vi "PSConverter.vi"(1 "Tbl Refnum":refnum<vi>, 2 "PROC":string[](array[string]), 3 "STATES":string[][](array[string]), 4 "Input claster":cluster{"TimeInState":u16, "cur_state":i8}[](array[cluster])) -> (0 "Current States":string[][](table))   [LabVIEW 2019]
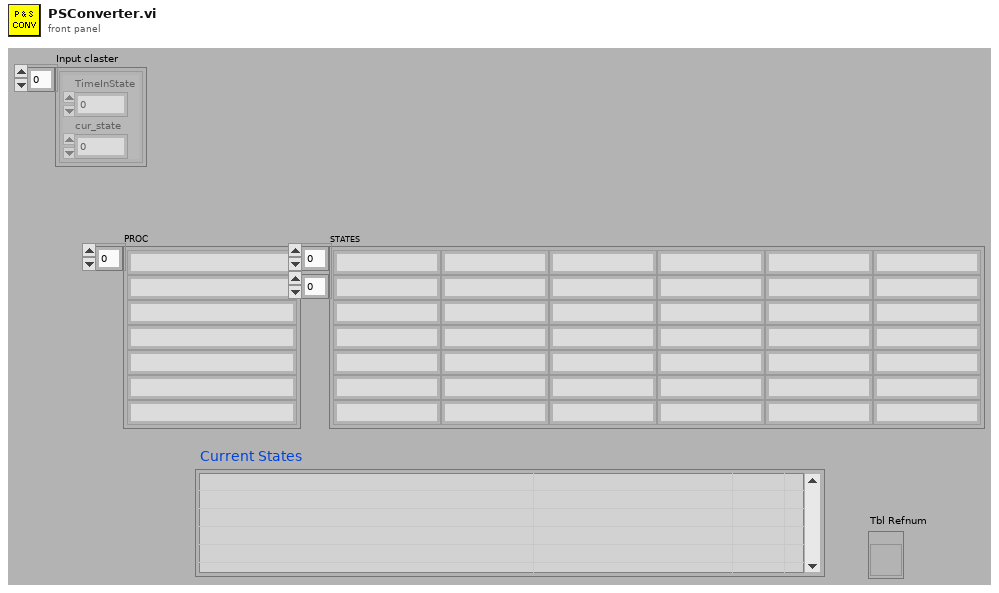
[diagram p1: front panel]
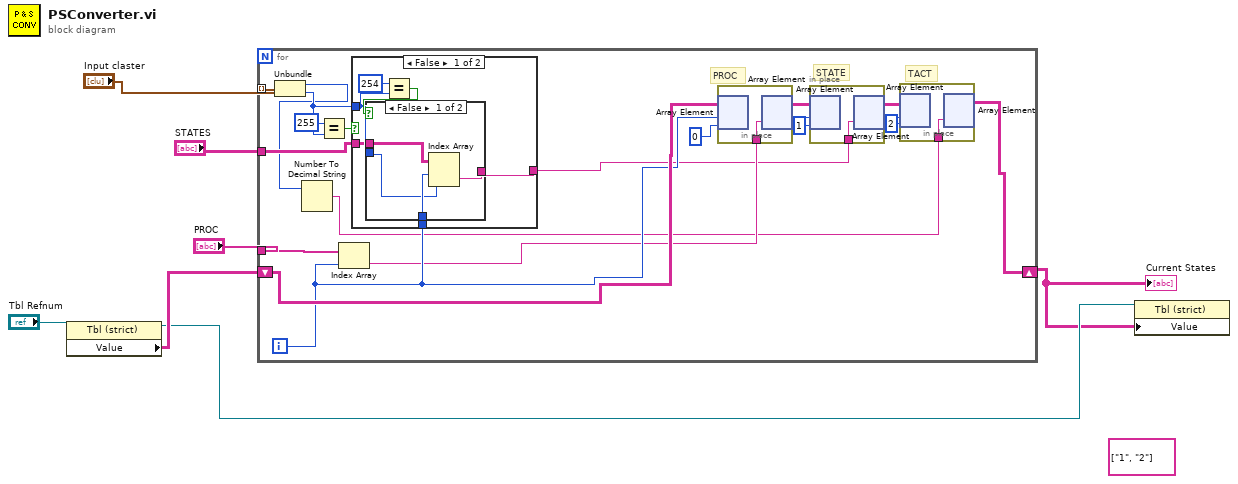
[diagram p0: block diagram]
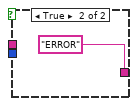
[diagram p2: hidden frame]
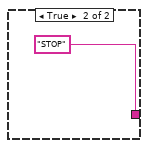
[diagram p3: hidden frame]
diagram:
  (unwired) string[][] [["1", "2"]] ("Value")
  n1 = property class="Tbl (strict)"(reference="Tbl Refnum") -> (reference out=w3:refnum<vi>, "Value"=w4:string[][])  [unwired: 1 in, 1 out]
  n2 = for {
    tunnel: "Input claster" -> [w27] mode=indexing
    tunnel: "PROC" -> [w23]
    tunnel: "STATES" -> [w22]
    shift-right: [w8] -> w1
    shift-left: w4 -> [w20]
    i -> [w19]
    # "TACT"
    # "STATE"
    # "PROC"
    n3 = Unbundle(w27) -> ("TimeInState"=w21:u16, "cur_state"=w24:i8)
    n4 = Number To Decimal String(number=w21) -> (decimal integer string=w9:string)  [unwired: 1 in]
    n5 = Equal?(x=u8 255, y=w24) -> (x = y?=w25:bool)
    n6 = Index Array(array=w23, index=w19) -> (element=w17:string)
    n7 = case shown="False" w25 {
      tunnel: w24 -> [w33 _]
      tunnel: [w31 "STOP"] -> w10
      tunnel: w19 -> [w34 _]
      tunnel: w22 -> [w32 _]
      frame False {
        n8 = Equal?(x=u8 254, y=w33) -> (x = y?=w35:bool)
        n9 = case shown="False" w35 {
          tunnel: [w37 "ERROR"] -> w31
          tunnel: w34 -> [w40 _]
          tunnel: w33 -> [w39 _]
          tunnel: w32 -> [w38 _]
          frame False {
            n10 = Index Array(array=w38, index (row)=w40, index (col)=w39) -> (element=w37:string)
          }
          frame True {
          }
        }
      }
      frame True {
      }
    }
    n11 = in-place {
      in-place-border: w17 -> [w30]
      n12 = in-place-array #1(w20, w19, 0 ("disabled index (col)")) -> ()  [unwired: 1 out]
      n13 = in-place-array #1(w30) -> (w14:string[][], w16:i32)  [unwired: 1 out]
    }
    n14 = in-place {
      in-place-border: w10 -> [w29]
      n15 = in-place-array #2(w14, w16, 1) -> ()  [unwired: 1 out]
      n16 = in-place-array #2(w29) -> (w13:string[][], w15:i32)  [unwired: 1 out]
    }
    n17 = in-place {
      in-place-border: w9 -> [w28]
      n18 = in-place-array #3(w13, w15, 2) -> ()  [unwired: 1 out]
      n19 = in-place-array #3(w28) -> (w8:string[][])  [unwired: 2 out]
    }
  }
  "Current States" <- w1
  n20 = property class="Tbl (strict)"(reference=w3, "Value"=w1) -> ()  [unwired: 1 in, 2 out]
